vi "Data Get Long (Polymorphic).vi"   [LabVIEW 2010]
uses:
  <vilib>/MDSplus/Library/MDSplus.lvlib
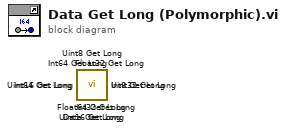
[diagram p0: block diagram]
diagram:
  n1 = call <vilib>:"Float64 Get Long.vi"() -> ()  [unwired: 9 in, 3 out]
  n2 = call <vilib>:"Float32 Get Long.vi"() -> ()  [unwired: 9 in, 3 out]
  n3 = call <vilib>:"Uint64 Get Long.vi"() -> ()  [unwired: 9 in, 3 out]
  n4 = call <vilib>:"Uint32 Get Long.vi"() -> ()  [unwired: 9 in, 3 out]
  n5 = call <vilib>:"Uint16 Get Long.vi"() -> ()  [unwired: 9 in, 3 out]
  n6 = call <vilib>:"Uint8 Get Long.vi"() -> ()  [unwired: 9 in, 3 out]
  n7 = call <vilib>:"Int64 Get Long.vi"() -> ()  [unwired: 9 in, 3 out]
  n8 = call <vilib>:"Int32 Get Long.vi"() -> ()  [unwired: 9 in, 3 out]
  n9 = call <vilib>:"Int16 Get Long.vi"() -> ()  [unwired: 9 in, 3 out]
  n10 = call <vilib>:"Int8 Get Long.vi"() -> ()  [unwired: 9 in, 3 out]
  n11 = call <vilib>:"Data Get Long.vi"() -> ()  [unwired: 9 in, 3 out]
